vi "GenerateCode.vi"(1 "Terms":T1[](array[typedef]), 3 "Diagram":refnum<vi>, 5 "XRef":refnum<vi>, 6 "State In":T4) -> (0 "Generated Code?":bool, 2 "State Out":T4, 4 "Reply":string[](array[string]))   [LabVIEW 2015, in "Async-Or-Show.xnode"]
doc: "This ability VI is called when it is time to define the execution behavior of your XNode via LabVIEW's scripting API. This VI is only called when you have previously informed LabVIEW that you need to script through a GenerateCode reply. Diagram is a reference to a diagram of a temporary VI. This diagram contains exactly one front panel terminal for each terminal of your XNode. Terms is an array of pairs of Term IDs and terminal references. LabVIEW will copy code scripted into this diagram into your XNode and connect everything to the correct terminals. The front panel terminals that are on this diagram are special in that they can only be on the top level diagram.\n \n Generate Code? is used to tell LabVIEW whether or not you want to copy the scripted diagram over. If there is an error and you wish not to commit the changes, then the old XNode behavior will be left unchanged. If you set Generate Code? to false, then this VI will be called again next time type propagation is run. Otherwise, it will not be called until you indicate that it should be through the reply on another ability VI.\n \n Because the diagram you are scripting into is separate from the VI containing the XNode instance, type propagation and the data manager will run on the temporary VI after each scripting call.\n \n You should not use the Copy scripting method to move code into the temporary VI. This will adversely affect the user's clipboard. You should use the Move scripting method instead.\n\nDefault behavior: None.\n\nThis ability does not provide UI and OS messages are not handled.\n\nSee also: ModifyCode"
uses:
  Async-Or-Show.xnode
  State.ctl
  <vilib>/Utility/miscctls.llb/LVRectTypeDef.ctl
  <vilib>/picture/picture.llb/imagedata.ctl
  <vilib>/XNodeSupport/XNodeTermIDPair.ctl
  <vilib>/XNodeSupport/XNodeTermRef.ctl
  <vilib>/XNodeSupport/XNodeString.ctl
  <vilib>/Erdos Miller/LV-Scripting/LV-Scripting.lvlib
  <vilib>/XNodeSupport/NI_XNodeSupport.lvlib
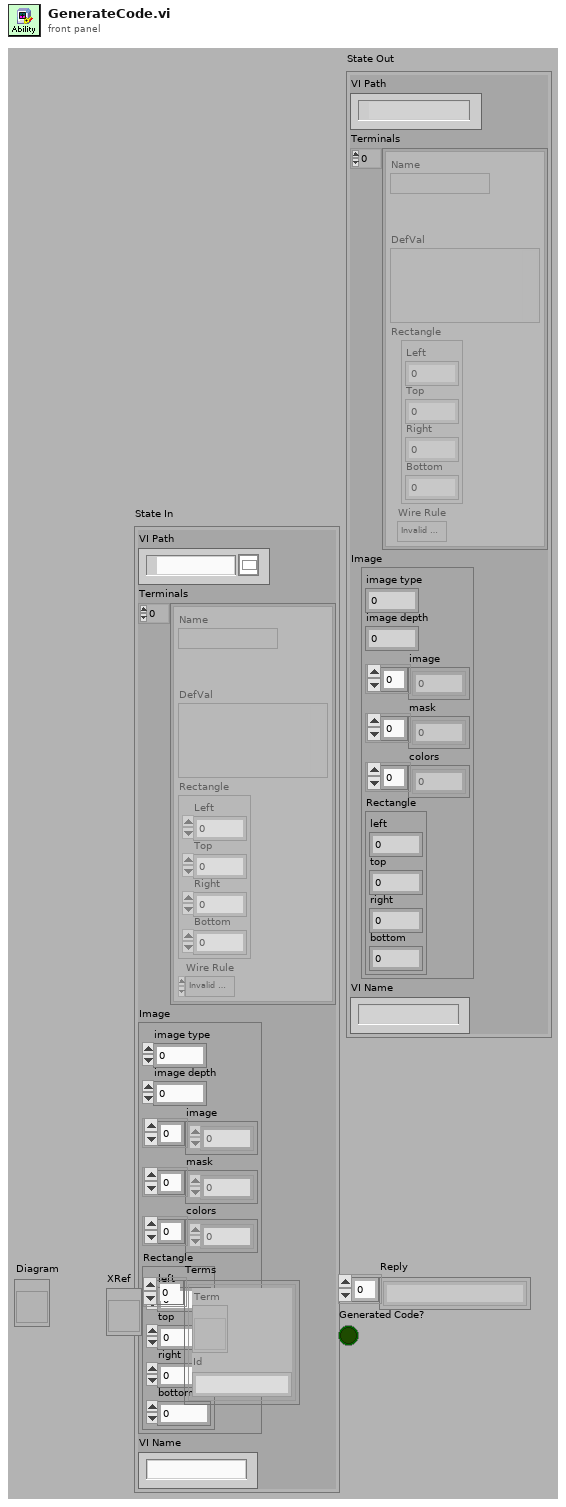
[diagram p1: front panel]
types:
  T1 = typedef "NI_XNodeSupport.lvlib/XNodeTermIDPair.ctl" = cluster{"Term":T2, "Id":T3}
  T2 = typedef "NI_XNodeSupport.lvlib/XNodeTermRef.ctl" = refnum<vi>
  T3 = typedef "NI_XNodeSupport.lvlib/XNodeString.ctl" = string
  T4 = typedef "Async-Or-Show.xnode/State.ctl" = cluster{"VI Path":path, "Terminals":cluster{"Name":string, "DefVal":variant, "Rectangle":T5, "Wire Rule":enum16{"Invalid Wire Rule", "Required", "Recommended", "Optional", "Dynamic Dispatch"}}[], "Image":T6, "VI Name":string}
  T5 = typedef "LVRectTypeDef.ctl" = cluster{"Left":i16, "Top":i16, "Right":i16, "Bottom":i16}
  T6 = typedef "imagedata.ctl" = cluster{"image type":i32, "image depth":i32, "image":u8[], "mask":u8[], "colors":u32[], "Rectangle":cluster{"left":i16, "top":i16, "right":i16, "bottom":i16}}
  T7 = cluster{"Name":string, "DefVal":variant, "Rectangle":T5, "Wire Rule":enum16{"Invalid Wire Rule", "Required", "Recommended", "Optional", "Dynamic Dispatch"}}[]
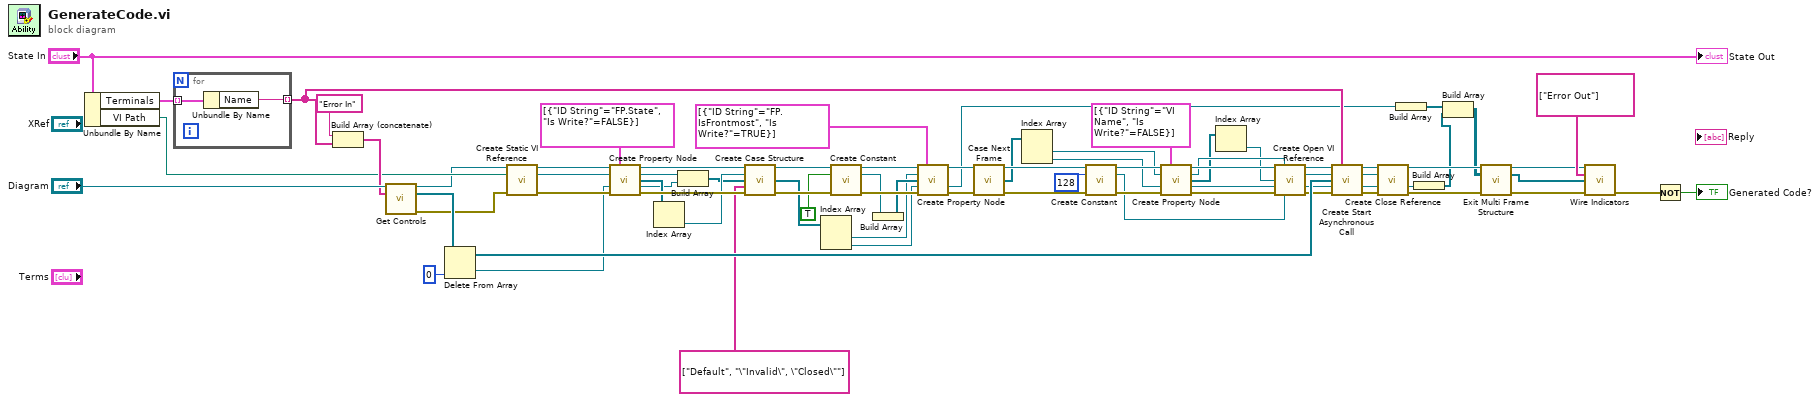
[diagram p0: block diagram]
diagram:
  n1 = Unbundle By Name("State In") -> ("Terminals"=w73:T7, "VI Path"=w68:path)
  n2 = for {
    tunnel: w73 -> [w77] mode=indexing
    tunnel: [w76] -> w57 mode=indexing
    n3 = Unbundle By Name(w77) -> ("Name"=w76:string)
  }
  n4 = Build Array (concatenate)("Error In" ("string"), w57) -> (w71:string[])
  n5 = call <vilib>:"Get Controls.vi"("Diagram in"="Diagram", "Control Names"=w71) -> ("Diagram out"=w67:refnum<vi>, "Control Terminals"=w70:refnum<vi>[], "error out"=w66:errorcluster)  [unwired: 11 in]
  n6 = Delete From Array(array=w70, index=0) -> (deleted portion=w9:refnum<vi>, array with subset deleted=w58:refnum<vi>[])  [unwired: 1 in]
  n7 = call <vilib>:"Create Static VI Reference.vi"("Diagram in"=w67, "VI Path"=w68, "error in (no error)"=w66) -> ("Diagram out"=w37:refnum<vi>, "Terminal"=w36:refnum<vi>, "error out"=w56:errorcluster)  [unwired: 10 in]
  n8 = call <vilib>:"Create Property Node.vi"("Diagram in"=w37, "Properties"=cluster{"ID String":string, "Is Write?":bool}[] [{"ID String"="FP.State", "Is Write?"=FALSE}], "reference"=w36, "error in"=w9, "error in (no error)"=w56) -> ("Diagram out"=w33:refnum<vi>, "reference out"=w29:refnum<vi>, "Outputs"=w31:refnum<vi>[], 10:"error out"=w23:refnum<vi>, 15:"error out"=w38:errorcluster)  [unwired: 6 in]
  n9 = Index Array(array=w31) -> (element=w30:refnum<vi>)  [unwired: 1 in]
  n10 = Build Array(w29, w23) -> (w28:refnum<vi>[])
  n11 = call <vilib>:"Create Case Structure.vi"("Diagram in"=w33, "Selector"=w30, "Inputs"=w28, "Frames"=string[] ["Default", "\"Invalid\", \"Closed\""], "error in (no error)"=w38) -> ("Selected Diagram"=w18:refnum<vi>, "Inputs"=w13:refnum<vi>[], "error out"=w34:errorcluster)  [unwired: 7 in, 1 out]
  n12 = Index Array(array=w13) -> (element #1=w12:refnum<vi>, element #2=w11:refnum<vi>)  [unwired: 2 in]
  n13 = call <vilib>:"Create Constant.vi"("Diagram in"=w18, "Type"=TRUE, "error in (no error)"=w34) -> ("Diagram out"=w17:refnum<vi>, "Terminal"=w15:refnum<vi>, "error out"=w19:errorcluster)  [unwired: 10 in]
  n14 = Build Array(w15) -> (w14:refnum<vi>[])
  n15 = call <vilib>:"Create Property Node.vi"("Diagram in"=w17, "Properties"=cluster{"ID String":string, "Is Write?":bool}[] [{"ID String"="FP.IsFrontmost", "Is Write?"=TRUE}], "reference"=w12, "Inputs"=w14, "error in"=w11, "error in (no error)"=w19) -> ("Diagram out"=w21:refnum<vi>, 10:"error out"=w10:refnum<vi>, 15:"error out"=w22:errorcluster)  [unwired: 5 in, 2 out]
  n16 = call <vilib>:"Case Next Frame.vi"("Diagram in"=w21, "error in (no error)"=w22) -> ("Selected Diagram"=w26:refnum<vi>, "Inputs"=w25:refnum<vi>[], "error out"=w27:errorcluster)  [unwired: 10 in, 1 out]
  n17 = Index Array(array=w25) -> (element #1=w24:refnum<vi>, element #2=w8:refnum<vi>)  [unwired: 2 in]
  n18 = call <vilib>:"Create Constant.vi"("Diagram in"=w26, "Type"=128, "error in (no error)"=w27) -> ("Diagram out"=w45:refnum<vi>, "Terminal"=w62:refnum<vi>, "error out"=w63:errorcluster)  [unwired: 10 in]
  n19 = call <vilib>:"Create Property Node.vi"("Diagram in"=w45, "Properties"=cluster{"ID String":string, "Is Write?":bool}[] [{"ID String"="VI Name", "Is Write?"=FALSE}], "reference"=w24, "error in"=w8, "error in (no error)"=w63) -> ("Diagram out"=w44:refnum<vi>, "reference out"=w42:refnum<vi>, "Outputs"=w41:refnum<vi>[], 10:"error out"=w39:refnum<vi>, 15:"error out"=w46:errorcluster)  [unwired: 6 in]
  n20 = Index Array(array=w41) -> (element=w40:refnum<vi>)  [unwired: 1 in]
  n21 = call <vilib>:"Create Open VI Reference.vi"("Diagram in"=w44, "type specifier"=w42, "vi path"=w40, "error in"=w39, "error in (no error)"=w46, "options"=w62) -> ("Diagram out"=w55:refnum<vi>, "vi reference"=w53:refnum<vi>, 10:"error out"=w52:refnum<vi>, 15:"error out"=w54:errorcluster)  [unwired: 6 in]
  n22 = call <vilib>:"Create Start Asynchronous Call.vi"("Diagram in"=w55, "Input Names"=w57, "reference"=w53, "Inputs"=w58, "error in"=w52, "error in (no error)"=w54) -> ("Diagram out"=w50:refnum<vi>, "reference out"=w49:refnum<vi>, 10:"error out"=w48:refnum<vi>, 15:"error out"=w59:errorcluster)  [unwired: 6 in]
  n23 = call <vilib>:"Create Close Reference.vi"("Diagram in"=w50, "application reference"=w49, "error in"=w48, "error in (no error)"=w59) -> ("Diagram out"=w6:refnum<vi>, 10:"error out"=w47:refnum<vi>, 15:"error out"=w51:errorcluster)  [unwired: 9 in]
  n24 = Build Array(w10) -> (w4:refnum<vi>[])
  n25 = Build Array(w47) -> (w3:refnum<vi>[])
  n26 = Build Array(w4, w3) -> (w2:refnum<vi>[][])
  n27 = call <vilib>:"Exit Multi Frame Structure.vi"("Diagram in"=w6, "Outputs"=w2, "error in (no error)"=w51) -> ("Diagram out"=w5:refnum<vi>, "Outputs"=w1:refnum<vi>[], "error out"=w7:errorcluster)  [unwired: 10 in]
  n28 = call <vilib>:"Wire Indicators.vi"("Diagram in"=w5, "Indicator Names"=string[] ["Error Out"], "Outputs"=w1, "error in (no error)"=w7) -> ("error out"=w60:errorcluster)  [unwired: 10 in, 1 out]
  n29 = Not(x=w60) -> (.not. x?=→"Generated Code?":bool)
  "State Out" <- "State In"
